vi "Discover Oven Model.vi"(10 "Model In":string) -> (2 "selection":bool)   [LabVIEW 2018]
panel:
  out "size(s)":i32
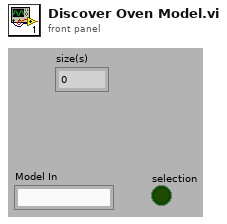
[diagram p1: front panel]
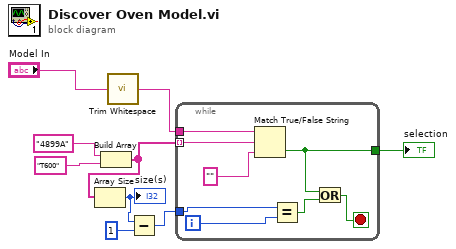
[diagram p0: block diagram]
diagram:
  n1 = Build Array("4899A" ("true string"), "T600" ("element")) -> (w7:string[])
  n2 = Array Size(array=w7) -> (size(s)=w6:i32)
  "size(s)" <- w6
  n3 = call <vilib>:"Trim Whitespace.vi"("string"="Model In") -> ("trimmed string"=w2:string)  [unwired: 1 in]
  n4 = Subtract(x=w6, y=1) -> (x-y=w4:i32)
  n5 = while {
    tunnel: w7 -> [w16] mode=indexing
    tunnel: w2 -> [w15]
    tunnel: [w14] -> w8
    tunnel: w4 -> [w10]
    i -> [w11]
    stop <- w13 stop-if-true
    n6 = Match True/False String(2:"" ("false string"), 3:w16, 4:w15) -> (0:w14:bool)  [unwired: 1 out]
    n7 = Equal?(x=w10, y=w11) -> (x = y?=w12:bool)
    n8 = Or(x=w14, y=w12) -> (x .or. y?=w13:bool)
  }
  "selection" <- w8
